vi "DrawStringWithSpecifiedFont.vi"(6 "underline? (F)":bool, 7 "position in":cluster{"left":u32, "top":u32}, 8 "error in (no error)":errorcluster, 9 "font":cluster{"name":string, "size":i16, "color":u32}, 10 "string":string, 11 "picture in":picture) -> (0 "error out":errorcluster, 3 "picture out":picture, 5 "position out":cluster{"left":u32, "top":u32})   [LabVIEW 2009, in "text.lvclass"]
uses:
  text.lvclass
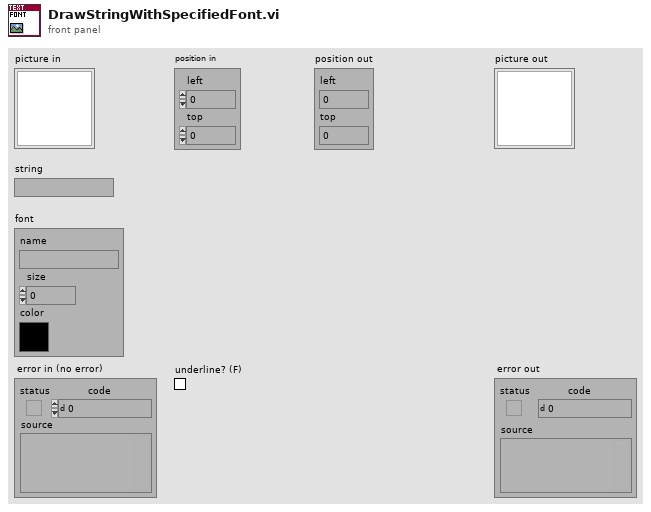
[diagram p1: front panel]
types:
  T1 = cluster{"Font Name:":string, "Size":i16, "Strikeout?":bool, "Italic?":bool, "Underline?":bool, "Outline?":bool, "Shadow?":bool, "Bold?":bool}
  T2 = enum16{"User-specified Font", "Application Font", "System Font", "Dialog Font"}
  T3 = cluster{"left":i16, "top":i16, "right":i16, "bottom":i16}
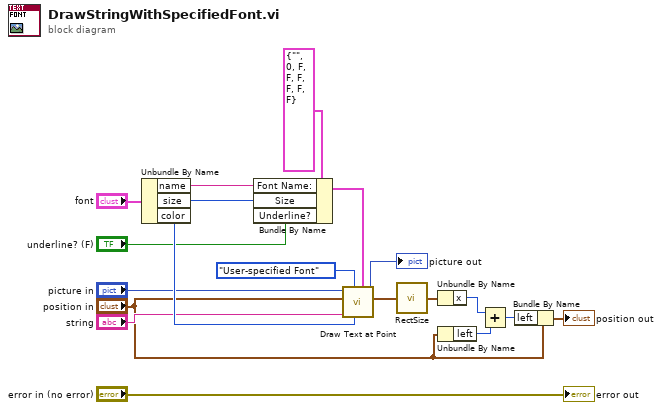
[diagram p0: block diagram]
diagram:
  n1 = Unbundle By Name("font") -> ("name"=w16:string, "size"=w15:i16, "color"=w14:u32)
  n2 = Bundle By Name(cluster=T1 {"Font Name:"="", "Size"=0, "Strikeout?"=FALSE, "Italic?"=FALSE, "Underline?"=FALSE, "Outline?"=FALSE, "Shadow?"=FALSE, "Bold?"=FALSE} ("[user-specified font]"), "Font Name:"=w16, "Size"=w15, "Underline?"="underline? (F)") -> (w17:T1)
  n3 = call <vilib>:"Draw Text at Point.vi"("[user-specified font]"=w17, "text color(black)"=w14, "desired font(Application)"=T2."User-specified Font", "text"="string", "origin"="position in", "picture"="picture in") -> ("text rect"=w10:T3, "new picture"=→"picture out":picture)  [unwired: 4 in]
  n4 = call <vilib>:"RectSize.vi"("rect"=w10) -> ("point"=w9:cluster{"x":i16, "y":i16})
  n5 = Unbundle By Name(w9) -> ("x"=w8:i16)
  n6 = Unbundle By Name("position in") -> ("left"=w6:u32)
  n7 = Add(x=w8, y=w6) -> (x+y=w5:u32)
  n8 = Bundle By Name(cluster="position in", "left"=w5) -> (→"position out":cluster{"left":u32, "top":u32})
  "error out" <- "error in (no error)"
